vi "VBD Main.vi"() -> ()   [LabVIEW 2017]
doc: "Use this template to build a simple state machine design pattern. Each state executes code and determines which state to transition to."
uses:
  controls/VBD State.ctl
  controls/VBD Data.ctl
  <vilib>/VirtualBench/_PS Configure Voltage Output2.vi
  <vilib>/VirtualBench/_FGEN Configure Standard Waveform20.vi
  <vilib>/VirtualBench/_MSO Configure Analog Channel28.vi
  <vilib>/VirtualBench/_MSO Configure Timing4.vi
  <vilib>/VirtualBench/VirtualBench.lvlib
panel:
  in  "Amplitude":dbl=2.0 caption="Amplitude (no change)" format="%#_gVpp"
  in  "Frequency":dbl=200.0 format="%#_gHz"
  in  "VirtualBench Device IO Control":tag="VB8012-308CBE9"
  out "Waveform Graph":waveform(dbl)[](graph)
  in  "Test Button":bool
  in  "Exit":bool
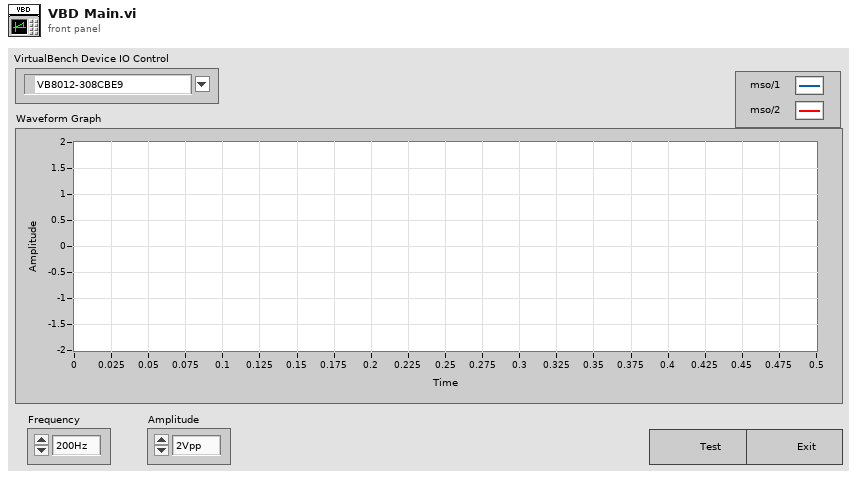
[diagram p1: front panel]
types:
  T1 = typedef "VBD Data.ctl" = cluster{"Boolean <Replace Me>":bool, "Steps":string, "Numeric <Replace Me>":dbl, "Output":waveform(dbl), "Filter Stages":waveform(dbl)[], "VB - FGEN Session":refnum<k21>, "VB - MSO Session":refnum<k21>, "VB - PS Session":refnum<k21>, "Log File Path":path}
  T2 = typedef "VBD State.ctl" = enum16{"Initialize", "Wait for Event", "Instructions", "VB - Setup", "VB - Acquire", "VB - Stop", "Log Data", "Exit"}
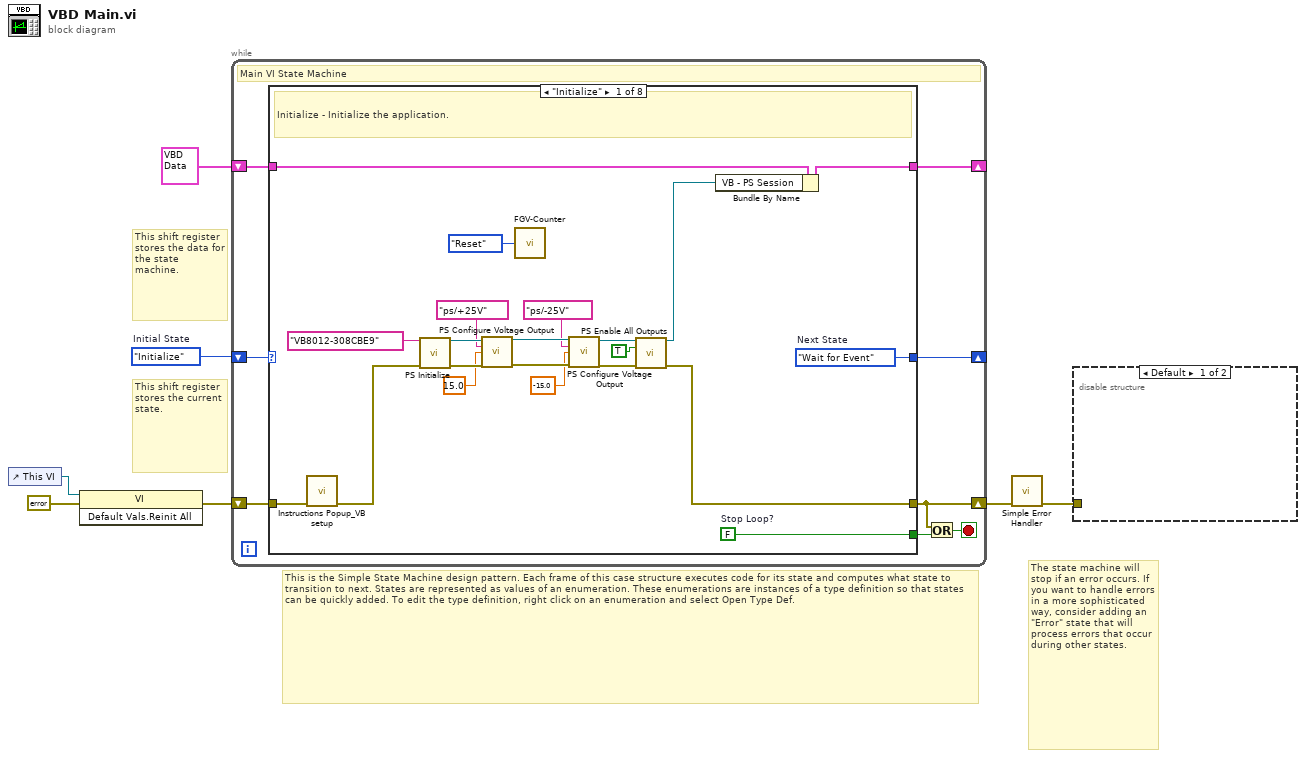
[diagram p0: block diagram]
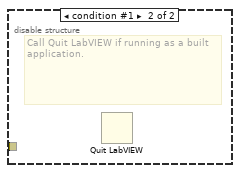
[diagram p2: hidden frame]
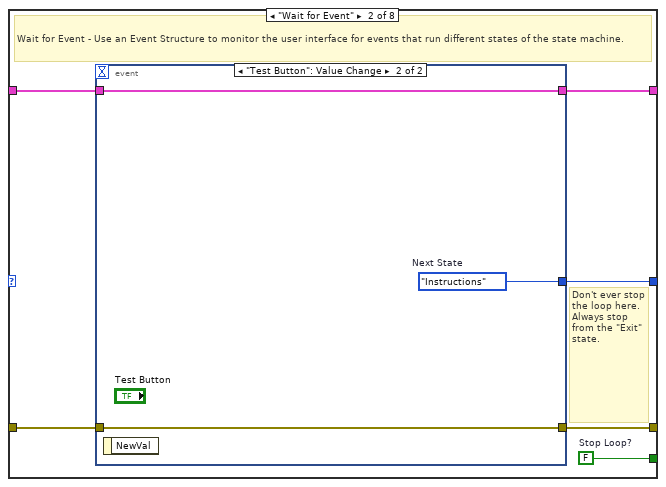
[diagram p3: hidden frame]
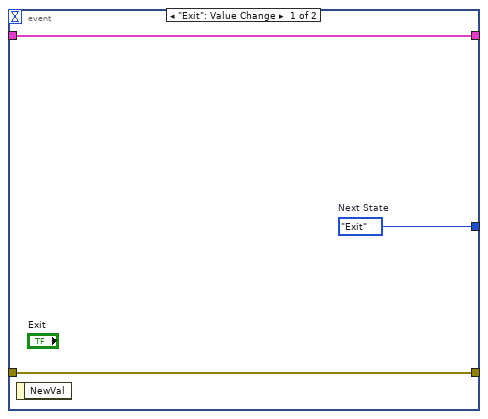
[diagram p4: hidden frame]
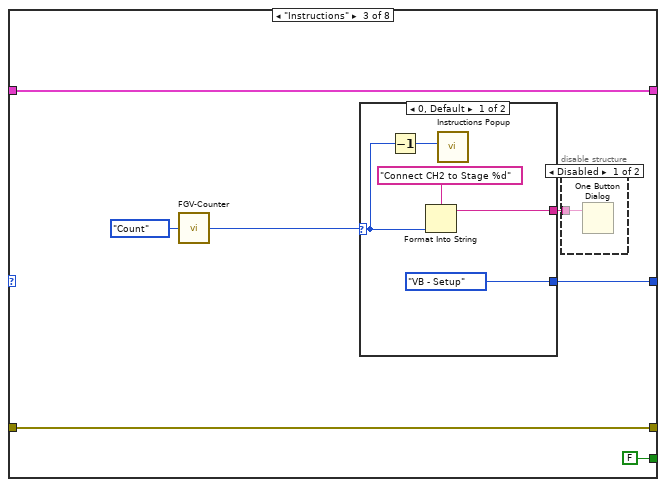
[diagram p5: hidden frame]
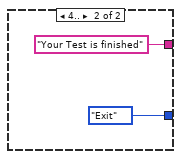
[diagram p7: hidden frame]
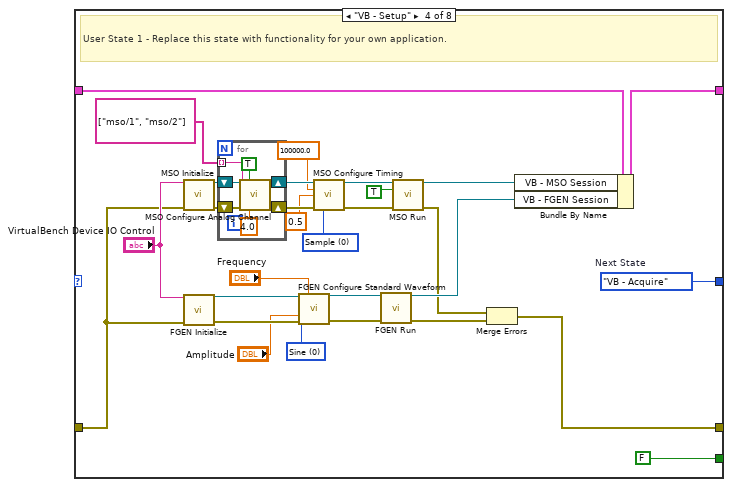
[diagram p8: hidden frame]
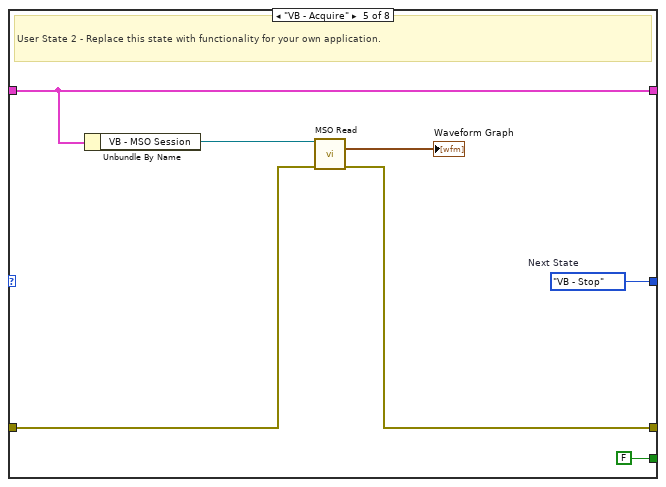
[diagram p9: hidden frame]
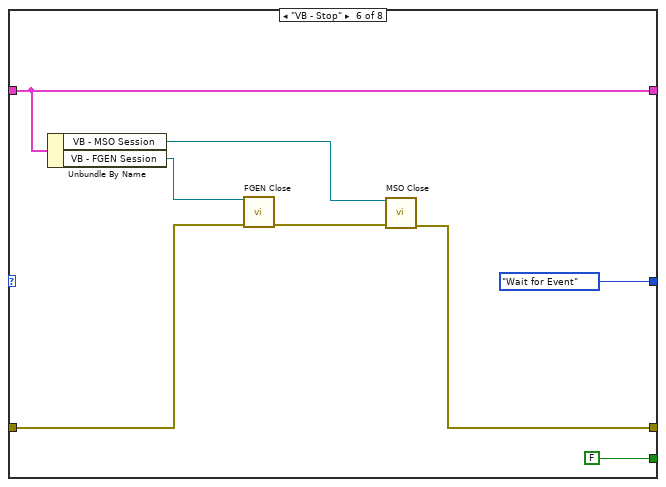
[diagram p10: hidden frame]
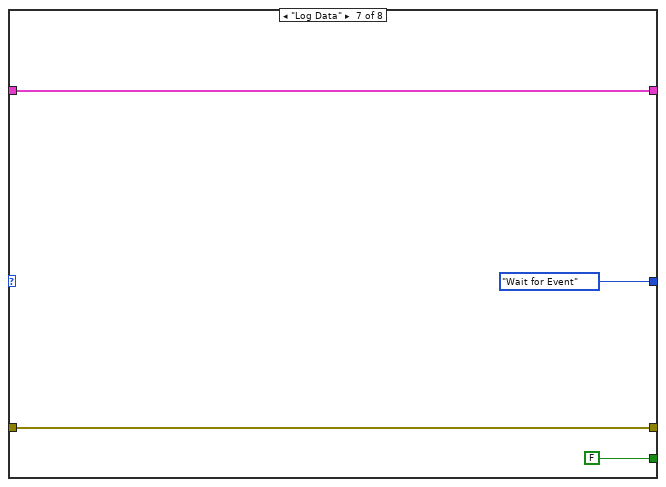
[diagram p11: hidden frame]
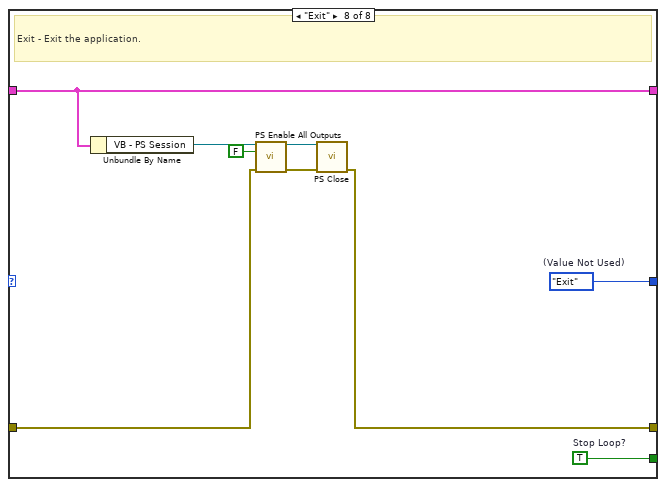
[diagram p12: hidden frame]
diagram:
  w7 = VBD_State."Initialize"  # Initial State
  # "The state machine will stop if an error occurs. If you want to handle errors in a more sophisticated way, consider adding an \"Error\" state that will process errors that occur during other states."
  # "This shift register stores the data for the state machine."
  # "This is the Simple State Machine design pattern. Each frame of this case structure executes code for its state and computes what state to transition to next. States are represented as values of an enumeration. These enumerations are instances of a type definition so that states can be quickly added. To edit the type definition, right click on an enumeration and select Open Type Def."
  # "This shift register stores the current state."
  n1 = control-ref of="This VI"() -> (w1:refnum<vi>)
  n2 = invoke class="VI" method="Default Vals.Reinit All"(reference=w1, error in=errorcluster {"status"=FALSE, "code"=0, "source"=""} ("error constant")) -> (error out=w2:errorcluster)  [unwired: 1 in, 2 out]
  n3 = while {
    shift-right: [w14] -> _
    shift-left: w7 -> [w15]
    shift-right: [w12] -> _
    shift-left: T1 {"Boolean <Replace Me>"=FALSE, "Steps"="", "Numeric <Replace Me>"=0.0, "Output"={"t0"=timestamp(0 s since 1904-01-01), "dt"=1.0, "Y"=[]}, "Filter Stages"=[], "VB - FGEN Session"="", "VB - MSO Session"="", "VB - PS Session"="", "Log File Path"=path ""} ("Data") -> [w13]
    shift-right: [w8] -> w4
    shift-left: w2 -> [w11]
    stop <- w9 stop-if-true
    # "Main VI State Machine"
    n4 = case shown="\"Initialize\"" w15 {
      tunnel: [w36 w42 w51 w92 w106 VBD_State."Wait for Event" ("(Value Not Used)") VBD_State."Wait for Event" ("(Value Not Used)") w127] -> w14
      tunnel: [w35 w41 FALSE ("Stop Loop?") FALSE ("Stop Loop?") FALSE ("Stop Loop?") FALSE ("Stop Loop?") FALSE ("Stop Loop?") w126] -> w10
      tunnel: w13 -> [w22 w40 w54 w89 w104 w114 w118 w125]
      tunnel: [w21 w39 w54 w90 w104 w114 w118 w125] -> w12
      tunnel: w11 -> [w19 w38 w55 w76 w101 w108 w117 w121]
      tunnel: [w18 w37 w55 w80 w100 w107 w117 w120] -> w8
      frame "Initialize" {
        w35 = FALSE  # Stop Loop?
        w36 = VBD_State."Wait for Event"  # Next State
        # "Initialize - Initialize the application."
        n5 = call "Instructions Popup_VB setup.vi"("error in (no error)"=w19) -> ("error out"=w16:errorcluster)  [unwired: 10 in]
        n6 = call <vilib>:"PS Initialize.vi"("Device Name"=tag "VB8012-308CBE9", "Error In"=w16) -> ("Instrument Handle Out"=w34:refnum<k21>, "Error Out"=w33:errorcluster)  [unwired: 12 in]
        n7 = call-poly <vilib>:"PS Configure Voltage Output.vi"("Instrument Handle In"=w34, "Channel"=tag "ps/+25V", "Voltage Level"=15.0, "Error In"=w33) -> ("Instrument Handle Out"=w32:refnum<k21>, "Error Out"=w31:errorcluster)  [unwired: 10 in]
        n8 = call "FGV-Counter.vi"("Option"=enum16{"Reset", "Count"}."Reset") -> ()  [unwired: 1 out]
        n9 = call-poly <vilib>:"PS Configure Voltage Output.vi"("Instrument Handle In"=w32, "Channel"=tag "ps/-25V", "Voltage Level"=-15.0, "Error In"=w31) -> ("Instrument Handle Out"=w30:refnum<k21>, "Error Out"=w29:errorcluster)  [unwired: 10 in]
        n10 = call <vilib>:"PS Enable All Outputs.vi"("Instrument Handle In"=w30, "Enable Outputs"=TRUE, "Error In"=w29) -> ("Instrument Handle Out"=w20:refnum<k21>, "Error Out"=w18:errorcluster)  [unwired: 11 in]
        n11 = Bundle By Name(cluster=w22, "VB - PS Session"=w20) -> (w21:T1)
      }
      frame "Wait for Event" {
        w41 = FALSE  # Stop Loop?
        # "Don't ever stop the loop here. Always stop from the \"Exit\" state."
        # "Wait for Event - Use an Event Structure to monitor the user interface for events that run different states of the state machine."
        n12 = event shown="[1] \"Test Button\": Value Change" {
          selector: _ -> [_ _]
          dyn-events: _ -> [_ _]
          timeout: _ -> [_ _]
          tunnel: [w45 w48] -> w42
          tunnel: w40 -> [w44 w47]
          tunnel: [w44 w47] -> w39
          tunnel: w38 -> [w43 w46]
          tunnel: [w43 w46] -> w37
          event "Exit": Value Change {
            w45 = VBD_State."Exit"  # Next State
            n13 = event-data() -> ()  [unwired: 1 in, 1 out]
          }
          event "Test Button": Value Change {
            w48 = VBD_State."Instructions"  # Next State
            n14 = event-data() -> ()  [unwired: 1 in, 1 out]
          }
        }
      }
      frame "Instructions" {
        n15 = call "FGV-Counter.vi"("Option"=enum16{"Reset", "Count"}."Count") -> ("output"=w49:i32)
        n16 = case shown="0, Default" w49 {
          selector: w49 -> [w58 _]
          tunnel: [VBD_State."VB - Setup" ("(Value Not Used)") VBD_State."Exit" ("(Value Not Used)")] -> w51
          tunnel: [w59 "Your Test is finished"] -> w50
          frame 0, Default {
            n17 = Decrement(x=w58) -> (x-1=w57:i32)
            n18 = Format Into String(format string="Connect CH2 to Stage %d" ("Running User State 1"), w58) -> (resulting string=w59:string)  [unwired: 2 in, 1 out]
            n19 = call "Instructions Popup.vi"("Ring"=w57) -> ()  [unwired: 11 in]
          }
          frame 4.. {
          }
        }
        n20 = disable-structure shown="Disabled" {
          disable-tunnel: w50 -> [w56 _]
          frame Disabled {
            n21 = One Button Dialog(message=w56) -> ()  [unwired: 1 in, 1 out]
          }
          frame Enabled {
          }
        }
      }
      frame "VB - Setup" {
        w69 = 0 items=["Sample", "Peak Detect"] ("Sampling Mode")
        w78 = 0 items=["Sine", "Square", "Triangle/Ramp", "DC"] ("Waveform Function")
        w92 = VBD_State."VB - Acquire"  # Next State
        # "User State 1 - Replace this state with functionality for your own application."
        n22 = call <vilib>:"MSO Initialize.vi"("Device Name"="VirtualBench Device IO Control", "Error In"=w76) -> ("Instrument Handle Out"=w68:refnum<k21>, "Error Out"=w67:errorcluster)  [unwired: 12 in]
        n23 = call <vilib>:"FGEN Initialize.vi"("Device Name"="VirtualBench Device IO Control", "Error In"=w76) -> ("Instrument Handle Out"=w87:refnum<k21>, "Error Out"=w86:errorcluster)  [unwired: 12 in]
        n24 = for {
          shift-right: [w96] -> w73
          shift-left: w68 -> [w95]
          shift-right: [w97] -> w77
          shift-left: w67 -> [w94]
          tunnel: tag[] ["mso/1", "mso/2"] -> [w93] mode=indexing
          n25 = call-poly <vilib>:"MSO Configure Analog Channel.vi"("Instrument Handle In"=w95, "Enable Channel"=TRUE, "Channel"=w93, "Error In"=w94, "Vertical Range"=4.0) -> ("Instrument Handle Out"=w96:refnum<k21>, "Error Out"=w97:errorcluster)  [unwired: 9 in]
        }
        n26 = call-poly <vilib>:"FGEN Configure Standard Waveform.vi"("Instrument Handle In"=w87, "Frequency"="Frequency", "Waveform Function"=w78, "Amplitude"="Amplitude", "Error In"=w86) -> ("Instrument Handle Out"=w85:refnum<k21>, "Error Out"=w84:errorcluster)  [unwired: 9 in]
        n27 = call-poly <vilib>:"MSO Configure Timing.vi"("Instrument Handle In"=w73, "Sample Rate"=100000.0, "Acquisition Time (s)"=0.5, "Error In"=w77, "Sampling Mode"=w69) -> ("Instrument Handle Out"=w72:refnum<k21>, "Error Out"=w74:errorcluster)  [unwired: 9 in]
        n28 = call <vilib>:"FGEN Run.vi"("Instrument Handle In"=w85, "Error In"=w84) -> ("Instrument Handle Out"=w83:refnum<k21>, "Error Out"=w81:errorcluster)  [unwired: 12 in]
        n29 = call <vilib>:"MSO Run.vi"("Instrument Handle In"=w72, "Auto Trigger"=TRUE, "Error In"=w74) -> ("Instrument Handle Out"=w88:refnum<k21>, "Error Out"=w82:errorcluster)  [unwired: 11 in]
        n30 = Merge Errors(w82, w81) -> (w80:errorcluster)
        n31 = Bundle By Name(cluster=w89, "VB - MSO Session"=w88, "VB - FGEN Session"=w83) -> (w90:T1)
      }
      frame "VB - Acquire" {
        w106 = VBD_State."VB - Stop"  # Next State
        # "User State 2 - Replace this state with functionality for your own application."
        n32 = Unbundle By Name(w104) -> ("VB - MSO Session"=w103:refnum<k21>)
        n33 = call <vilib>:"MSO Read.vi"("Instrument Handle In"=w103, "Error In"=w101) -> ("Analog Waveforms"=→"Waveform Graph":waveform(dbl)[], "Error Out"=w100:errorcluster)  [unwired: 8 in, 4 out]
      }
      frame "VB - Stop" {
        n34 = Unbundle By Name(w114) -> ("VB - MSO Session"=w113:refnum<k21>, "VB - FGEN Session"=w112:refnum<k21>)
        n35 = call <vilib>:"FGEN Close.vi"("Instrument Handle In"=w112, "Error In"=w108) -> ("Error Out"=w109:errorcluster)  [unwired: 13 in]
        n36 = call <vilib>:"MSO Close.vi"("Instrument Handle In"=w113, "Error In"=w109) -> ("Error Out"=w107:errorcluster)  [unwired: 13 in]
      }
      frame "Log Data" {
      }
      frame "Exit" {
        w126 = TRUE  # Stop Loop?
        w127 = VBD_State."Exit"  # (Value Not Used)
        # "Exit - Exit the application."
        n37 = Unbundle By Name(w125) -> ("VB - PS Session"=w124:refnum<k21>)
        n38 = call <vilib>:"PS Enable All Outputs.vi"("Instrument Handle In"=w124, "Enable Outputs"=FALSE, "Error In"=w121) -> ("Instrument Handle Out"=w123:refnum<k21>, "Error Out"=w119:errorcluster)  [unwired: 11 in]
        n39 = call <vilib>:"PS Close.vi"("Instrument Handle In"=w123, "Error In"=w119) -> ("Error Out"=w120:errorcluster)  [unwired: 13 in]
      }
    }
    n40 = Or(x=w8, y=w10) -> (x .or. y?=w9:bool)
  }
  n41 = call <vilib>:"Simple Error Handler.vi"("error in (no error)"=w4) -> ("error out"=w3:errorcluster)  [unwired: 4 in, 4 out]
  n42 = disable-structure shown="Default" {
    disable-tunnel: w3 -> [_ _]
    frame condition #0 (active) {
    }
    frame condition #1 {
      # "Call Quit LabVIEW if running as a built application."
      n43 = Quit LabVIEW() -> ()  [unwired: 1 in]
    }
  }
